vi "Create Freq Input.vi"(8 "error in (no error)":errorcluster, 10 "Params":variant, 11 "NI Counter Input in":refnum<class "NI Counter Input.lvclass">) -> (0 "error out":errorcluster, 3 "NI Counter Input out":refnum<class "NI Counter Input.lvclass">)   [LabVIEW 2020, in "NI DAQmx.lvlib" / "NI Counter Input.lvclass"]
uses:
  NI Counter Input.lvclass
  D:/WSGitHub/RTFWK/Realization/NI DAQmx Base/NI DAQmx Base.lvclass
  TypeDefs/Pulse input.ctl
  <vilib>/DAQmx/create/channels.llb/DAQmx Create Channel (CI-Frequency).vi
  <vilib>/DAQmx/configure/timing.llb/DAQmx Timing (Implicit).vi
  <resource>/objmgr/daqmx.rc
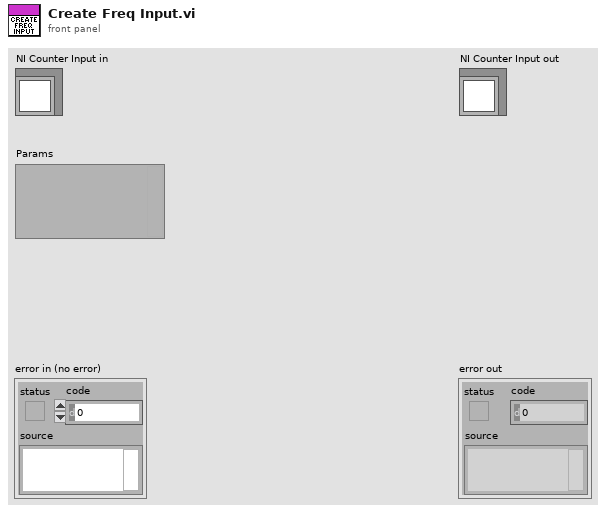
[diagram p1: front panel]
types:
  T1 = typedef "Pulse input.ctl" = cluster{"channel":string, "min_freq":dbl, "max_freq":dbl, "measurement_time":dbl, "samples":i32}
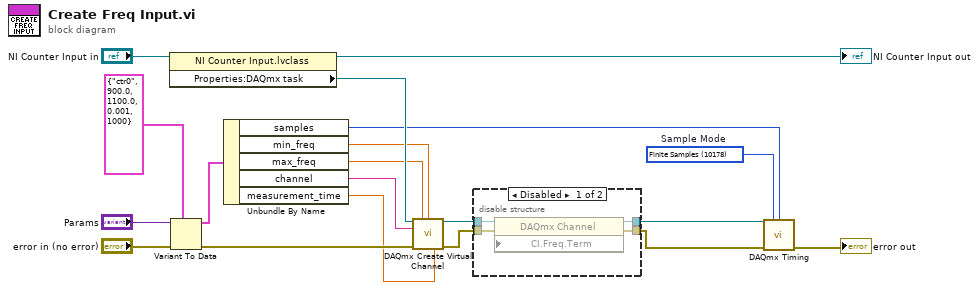
[diagram p0: block diagram]
diagram:
  w15 = 10178 items=["Finite Samples"=10178, "Continuous Samples"=10123, "Hardware Timed Single Point"=12522]  # Sample Mode
  n1 = property class="NI Counter Input.lvclass"(reference="NI Counter Input in") -> (reference out=→"NI Counter Input out":refnum<class "NI Counter Input.lvclass">, "Properties:DAQmx task"=w9:refnum<k21>)  [unwired: 1 in, 1 out]
  n2 = Variant To Data(error in="error in (no error)", type=T1 {"channel"="ctr0", "min_freq"=900.0, "max_freq"=1100.0, "measurement_time"=0.001, "samples"=1000}, Variant="Params") -> (data=w7:T1, error out=w11:errorcluster)
  n3 = Unbundle By Name(w7) -> ("samples"=w6:i32, "min_freq"=w3:dbl, "max_freq"=w4:dbl, "channel"=w5:string, "measurement_time"=w2:dbl)
  n4 = call-poly <vilib>:"DAQmx Create Virtual Channel.vi"("task in"=w9, "maximum value"=w4, "minimum value"=w3, "counter"=w5, "error in"=w11, "measurement time"=w2) -> ("task out"=w13:refnum<k21>, "error out"=w12:errorcluster)  [unwired: 8 in]
  n5 = disable-structure shown="Disabled" {
    disable-tunnel: [w23 w24] -> w1
    disable-tunnel: [w22 w25] -> w14
    disable-tunnel: w13 -> [w21 w25]
    disable-tunnel: w12 -> [w20 w24]
    frame Disabled {
      n6 = property class="DAQmx Channel" props=["CI.Freq.Term"](reference=w21, error in=w20) -> (reference out=w22:refnum<k21>, error out=w23:errorcluster)  [unwired: 1 in]
    }
    frame Enabled {
    }
  }
  n7 = call-poly <vilib>:"DAQmx Timing.vi"("task/channels in"=w14, "sample mode"=w15, "samples per channel"=w6, "error in"=w1) -> ("error out"=→"error out":errorcluster)  [unwired: 10 in, 1 out]
